vi "GetADCsection.vi"(8 "error in (no error)":errorcluster caption="에러 입력(에러 없음)", 10 "SectionMap":T1, 11 "ABFFIO 입력":refnum<class "ABFFIO.lvclass">) -> (0 "error out":errorcluster caption="에러 출력", 3 "ABFFIO 출력":refnum<class "ABFFIO.lvclass">)   [LabVIEW 2017, in "ABFFIO.lvclass"]
uses:
  ABFFIO.lvclass
  ABFFIO.lvclass/ABFFIO.ctl
panel:
  out "TelegraphEnable":u8
  out "TelegraphAdditGain":sgl
  out "SignalOffset":sgl
  out "SignalGain":sgl
  out "IntrumentOffset":sgl
  out "InstrumentScaleFactor":sgl
  out "ADCDisplayOffset":sgl
  out "ADCDisplayAmplification":sgl
  out "ADCProgrammableGain":sgl
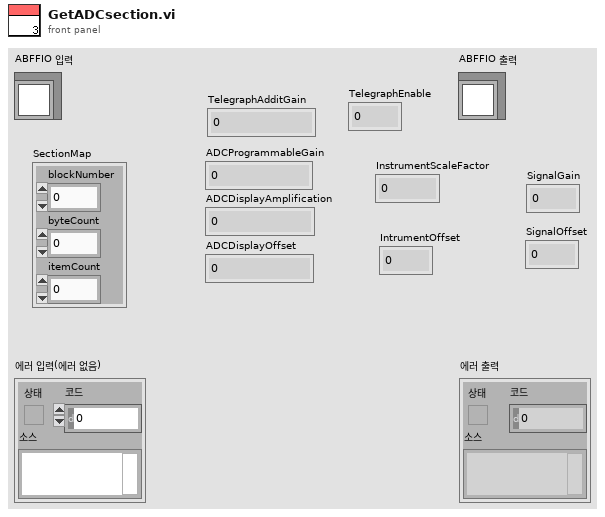
[diagram p1: front panel]
types:
  T1 = cluster{"blockNumber":u32, "byteCount":u32, "itemCount":u32}
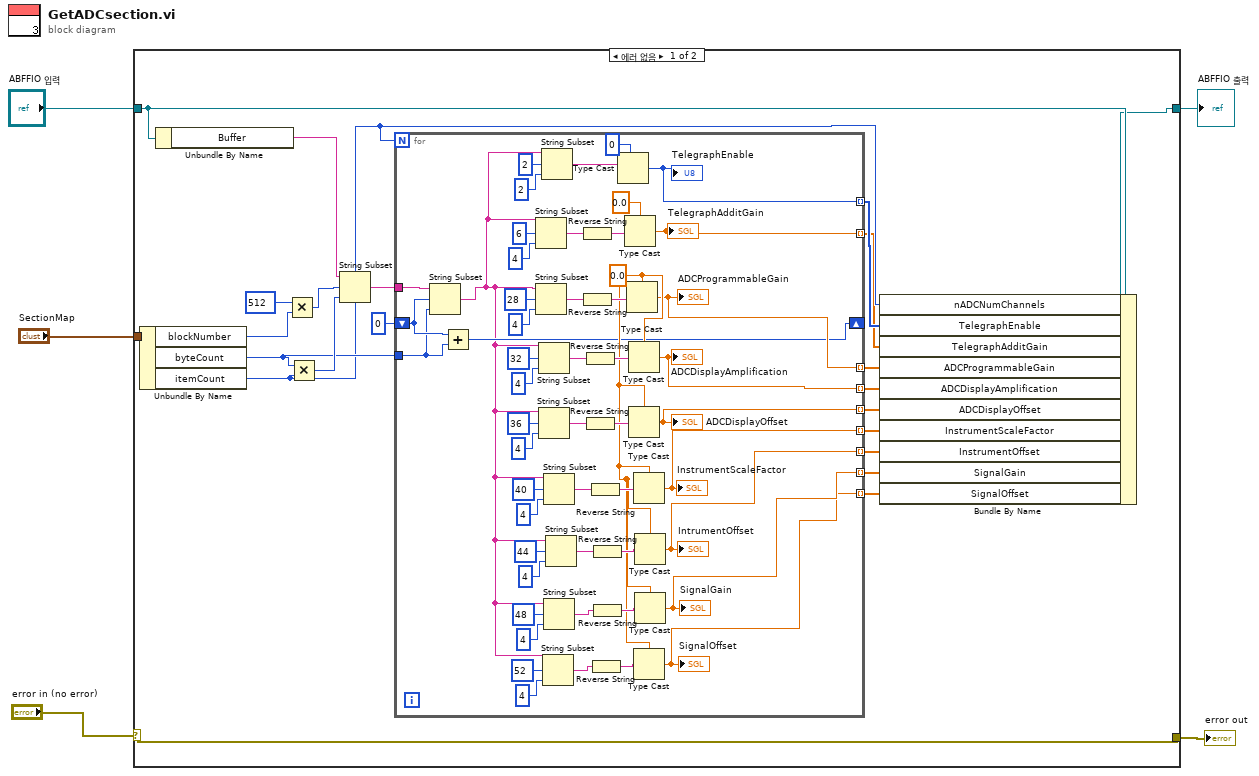
[diagram p0: block diagram]
diagram:
  n1 = case shown="에러 없음" "error in (no error)" {
    selector: "error in (no error)" -> [w27 w81]
    tunnel: [w27 w81] -> w4
    tunnel: [w11 w80] -> w2
    tunnel: "ABFFIO 입력" -> [w19 w80]
    tunnel: "SectionMap" -> [w25 _]
    frame No Error {
      n2 = Unbundle By Name(w25) -> ("blockNumber"=w24:u32, "byteCount"=w10:u32, "itemCount"=w8:u32)
      n3 = Unbundle By Name(w19) -> ("Buffer"=w26:string)
      n4 = Multiply(x=u32 512, y=w24) -> (x*y=w22:u32)
      n5 = Multiply(x=w10, y=w8) -> (x*y=w21:u32)
      n6 = String Subset(string=w26, offset (0)=w22, length (rest)=w21) -> (substring=w20:string)
      n7 = for {
        N: w8 -> [_]
        tunnel: w20 -> [w43]
        tunnel: [w50] -> w18 mode=indexing
        tunnel: [w49] -> w17 mode=indexing
        tunnel: [w48] -> w16 mode=indexing
        tunnel: [w47] -> w15 mode=indexing
        tunnel: [w46] -> w14 mode=indexing
        tunnel: [w45] -> w13 mode=indexing
        tunnel: [w44] -> w12 mode=indexing
        tunnel: w10 -> [w41]
        shift-right: [w40] -> _
        shift-left: u32 0 ("x") -> [w42]
        tunnel: [w29] -> w7 mode=indexing
        tunnel: [w28] -> w6 mode=indexing
        w51 = sgl 0.0 ("길이(나머지)")
        n8 = String Subset(string=w43, offset (0)=w42, length (rest)=w41) -> (substring=w32:string)
        n9 = Add(x=w42, y=w41) -> (x+y=w40:u32)
        n10 = String Subset(string=w32, offset (0)=6 ("오프셋(0)"), length (rest)=4 ("길이(나머지)")) -> (substring=w37:string)
        n11 = String Subset(string=w32, offset (0)=28 ("오프셋(0)"), length (rest)=4 ("길이(나머지)")) -> (substring=w77:string)
        n12 = String Subset(string=w32, offset (0)=32 ("오프셋(0)"), length (rest)=4 ("길이(나머지)")) -> (substring=w74:string)
        n13 = String Subset(string=w32, offset (0)=36 ("오프셋(0)"), length (rest)=4 ("길이(나머지)")) -> (substring=w69:string)
        n14 = String Subset(string=w32, offset (0)=2 ("오프셋(0)"), length (rest)=2 ("길이(나머지)")) -> (substring=w31:string)
        n15 = String Subset(string=w32, offset (0)=52 ("오프셋(0)"), length (rest)=4 ("길이(나머지)")) -> (substring=w53:string)
        n16 = String Subset(string=w32, offset (0)=40 ("오프셋(0)"), length (rest)=4 ("길이(나머지)")) -> (substring=w66:string)
        n17 = String Subset(string=w32, offset (0)=48 ("오프셋(0)"), length (rest)=4 ("길이(나머지)")) -> (substring=w58:string)
        n18 = String Subset(string=w32, offset (0)=44 ("오프셋(0)"), length (rest)=4 ("길이(나머지)")) -> (substring=w61:string)
        n19 = Reverse String(1:w37) -> (0:w36:string)
        n20 = Reverse String(1:w77) -> (0:w76:string)
        n21 = Reverse String(1:w74) -> (0:w75:string)
        n22 = Reverse String(1:w69) -> (0:w68:string)
        n23 = Reverse String(1:w66) -> (0:w67:string)
        n24 = Reverse String(1:w53) -> (0:w52:string)
        n25 = Reverse String(1:w61) -> (0:w60:string)
        n26 = Reverse String(1:w58) -> (0:w59:string)
        n27 = Type Cast(type=u8 0 ("길이(나머지)"), x=w31) -> (*(type *) &x=w29:u8)
        "TelegraphEnable" <- w29
        n28 = Type Cast(type=sgl 0.0 ("길이(나머지)"), x=w36) -> (*(type *) &x=w28:sgl)
        "TelegraphAdditGain" <- w28
        n29 = Type Cast(type=w51, x=w76) -> (*(type *) &x=w50:sgl)
        "ADCProgrammableGain" <- w50
        n30 = Type Cast(type=w51, x=w75) -> (*(type *) &x=w49:sgl)
        "ADCDisplayAmplification" <- w49
        n31 = Type Cast(type=w51, x=w68) -> (*(type *) &x=w48:sgl)
        "ADCDisplayOffset" <- w48
        n32 = Type Cast(type=w51, x=w67) -> (*(type *) &x=w47:sgl)
        "InstrumentScaleFactor" <- w47
        n33 = Type Cast(type=w51, x=w52) -> (*(type *) &x=w44:sgl)
        "SignalOffset" <- w44
        n34 = Type Cast(type=w51, x=w60) -> (*(type *) &x=w46:sgl)
        "IntrumentOffset" <- w46
        n35 = Type Cast(type=w51, x=w59) -> (*(type *) &x=w45:sgl)
        "SignalGain" <- w45
      }
      n36 = Bundle By Name(cluster=w19, "nADCNumChannels"=w8, "TelegraphEnable"=w7, "TelegraphAdditGain"=w6, "ADCProgrammableGain"=w18, "ADCDisplayAmplification"=w17, "ADCDisplayOffset"=w16, "InstrumentScaleFactor"=w15, "InstrumentOffset"=w14, "SignalGain"=w13, "SignalOffset"=w12) -> (w11:refnum<class "ABFFIO.lvclass">)
    }
    frame Error {
    }
  }
  "error out" <- w4
  "ABFFIO 출력" <- w2
